vi "UpdateBufferForMultiListBoxIfNecessary.vi"(7 "control refs":T2, 8 "error in":errorcluster, 9 "Buffer Configuration":T3, 10 "TDMS File Viewer Configuration":T3, 11 "TDMS descriptor array":T1(array[cluster])) -> (0 "error out":errorcluster, 1 "BufferConfig out":T3, 3 "TDMS descriptor array out":T1(array[cluster]))   [LabVIEW 2015]
uses:
  <vilib>/Utility/tdmsutil.llb/fileViewerConfigData.ctl
panel:
  in  "tdms file in":refnum<k34>
  out "tdms file out":refnum<k34>
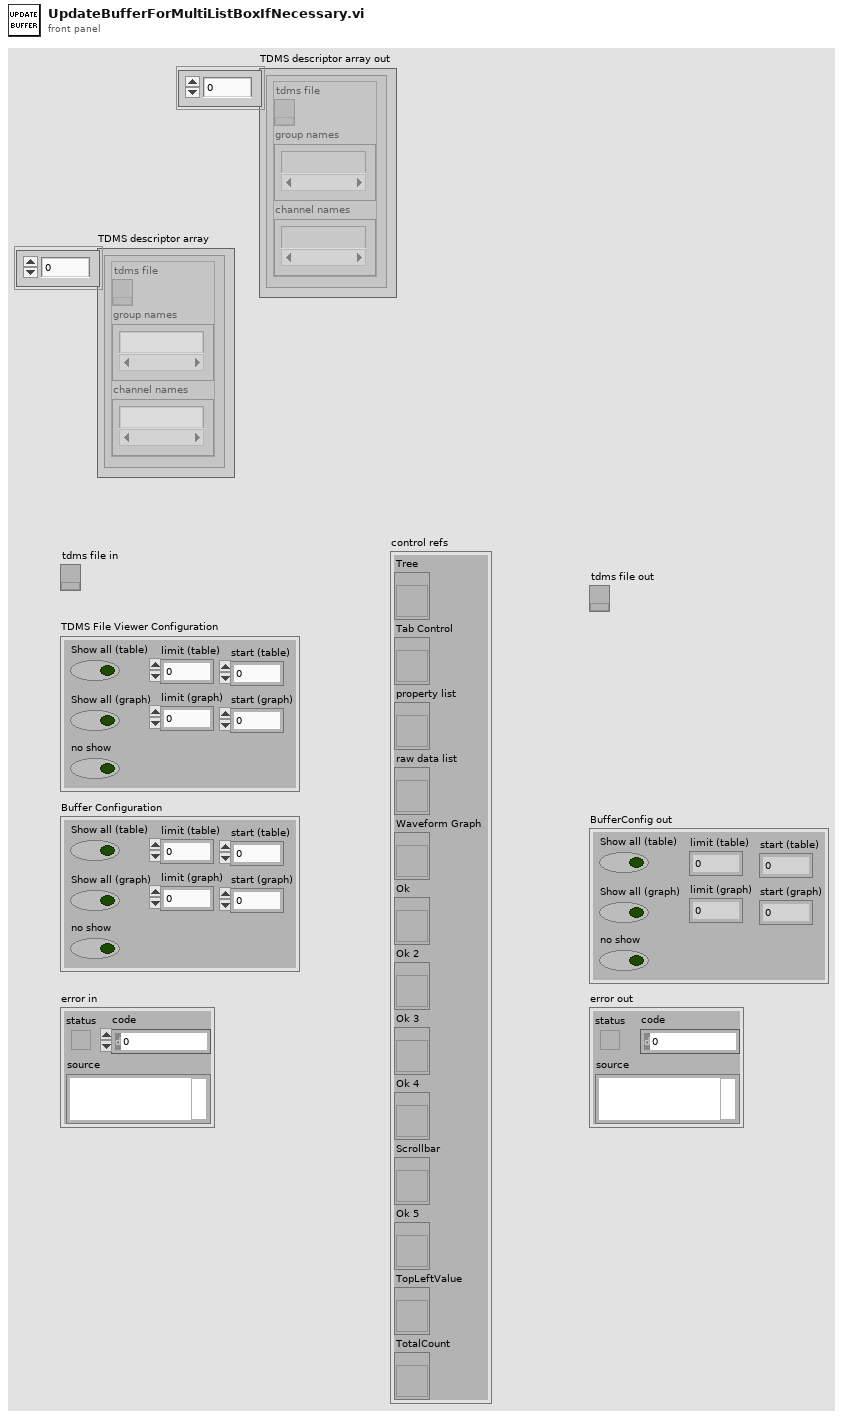
[diagram p1: front panel]
types:
  T1 = cluster{"tdms file ":refnum<k34>, "group names":string[], "channel names":string[]}[]
  T2 = cluster{"Tree":refnum<vi>, "Tab Control":refnum<vi>, "property list":refnum<vi>, "raw data list":refnum<vi>, "Waveform Graph":refnum<vi>, "Ok":refnum<vi>, "Ok 2":refnum<vi>, "Ok 3":refnum<vi>, "Ok 4":refnum<vi>, "Scrollbar":refnum<vi>, "Ok 5":refnum<vi>, "TopLeftValue":refnum<vi>, "TotalCount":refnum<vi>}
  T3 = typedef "fileViewerConfigData.ctl" = cluster{"Show all (table)":bool, "Show all (graph)":bool, "limit (table)":u64, "limit (graph)":u64, "no show":bool, "start (table)":u64, "start (graph)":u64}
  T4 = typedef "LVRowAndColumnUnsignedTypeDef.ctl" = cluster{"Row":u32, "Column":u32}
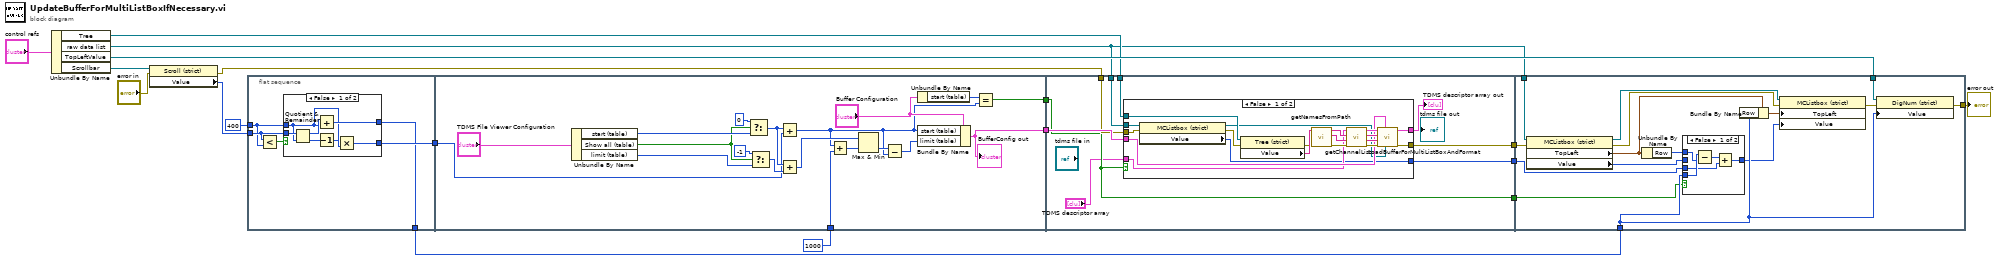
[diagram p0: block diagram]
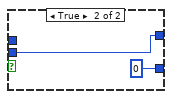
[diagram p2: hidden frame]
diagram:
  n1 = Unbundle By Name("control refs") -> ("Tree"=w8:refnum<vi>, "raw data list"=w7:refnum<vi>, "TopLeftValue"=w16:refnum<vi>, "Scrollbar"=w18:refnum<vi>)
  n2 = property on="Property Node" class="Scroll (strict)"(reference=w18, error in="error in") -> (error out=w9:errorcluster, "Value"=w14:u64)  [unwired: 1 out]
  n3 = flat-sequence {
    tunnel: [w22] -> w15
    tunnel: w14 -> [w21]
    tunnel: [w20] -> w13
    tunnel: u64 400 ("y") -> [w19]
    tunnel: w15 -> [w37]
    tunnel: [w36] -> w12
    tunnel: [w35] -> w11
    tunnel: u64 1000 ("y") -> [w33]
    tunnel: w12 -> [w55]
    tunnel: w11 -> [w60]
    tunnel: [w59] -> w10
    tunnel: w9 -> [w58]
    tunnel: w8 -> [w57]
    tunnel: w7 -> [w56]
    tunnel: [w55] -> w3
    tunnel: [w54] -> w2
    tunnel: w7 -> [w92]
    tunnel: w13 -> [w88]
    tunnel: w16 -> [w91]
    tunnel: w10 -> [w90]
    tunnel: [w89] -> w6
    tunnel: w3 -> [w87]
    tunnel: w2 -> [w86]
    frame #0 {
      n4 = Less?(x=w21, y=w19) -> (x < y?=w23:bool)
      n5 = case shown="False" w23 {
        tunnel: w21 -> [w30 w32]
        tunnel: [w28 w32] -> w20
        tunnel: [w27 u64 0] -> w22
        tunnel: w19 -> [w26 _]
        frame False {
          n6 = Quotient & Remainder(x=w30, y=w26) -> (x-y*floor(x/y)=w29:u64, floor(x/y)=w25:u64)
          n7 = Add(x=w29, y=w26) -> (x+y=w28:u64)
          n8 = Decrement(x=w25) -> (x-1=w24:u64)
          n9 = Multiply(x=w24, y=w26) -> (x*y=w27:u64)
        }
        frame True {
        }
      }
    }
    frame #1 {
      n10 = Unbundle By Name("TDMS File Viewer Configuration") -> ("start (table)"=w45:u64, "Show all (table)"=w38:bool, "limit (table)"=w44:u64)
      n11 = Select(t=u64 0, s=w38, f=w45) -> (s? t:f=w43:u64)
      n12 = Select(t=i64 -1, s=w38, f=w44) -> (s? t:f=w42:u64)
      n13 = Add(x=w43, y=w37) -> (x+y=w34:u64)
      n14 = Add(x=w43, y=w42) -> (x+y=w41:u64)
      n15 = Add(x=w34, y=w33) -> (x+y=w50:u64)
      n16 = Max & Min(x=w41, y=w50) -> (min(x,y)=w49:u64)  [unwired: 1 out]
      n17 = Subtract(x=w49, y=w34) -> (x-y=w48:u64)
      n18 = Unbundle By Name("Buffer Configuration") -> ("start (table)"=w46:u64)
      n19 = Bundle By Name(cluster="Buffer Configuration", "start (table)"=w34, "limit (table)"=w48) -> (w35:T3)
      "BufferConfig out" <- w35
      n20 = Equal?(x=w46, y=w34) -> (x = y?=w36:bool)
    }
    frame #2 {
      n21 = case shown="False" w55 {
        tunnel: [w75 w81] -> w59
        tunnel: [w70 w80] -> w52
        tunnel: w60 -> [w69 _]
        tunnel: w57 -> [w68 _]
        tunnel: w58 -> [w64 w81]
        tunnel: w56 -> [w65 _]
        tunnel: "TDMS descriptor array" -> [w66 w80]
        tunnel: [w61 _] -> w54
        frame False {
          n22 = property on="Property Node" class="MCListbox (strict)"(reference=w65, error in=w64) -> (reference out=w63:refnum<vi>, error out=w62:errorcluster, "Value"=w61:i32)
          n23 = property class="Tree (strict)"(reference=w68, error in=w62) -> (error out=w67:errorcluster, "Value"=w79:string)  [unwired: 1 out]
          n24 = call "getNamesFromPath.vi"("error in (no error)"=w67, "tree path"=w79) -> ("error out"=w78:errorcluster, "channel"=w76:string, "group"=w77:string)  [unwired: 1 in, 2 out]
          n25 = call "getChannelList.vi"("error in (no error)"=w78, "channel names"=w76, "group name"=w77, "TDMS descriptor array"=w66) -> ("error out"=w74:errorcluster, "channel names out"=w73:string[], "group names out"=w72:string[], "TDMS descriptor array out"=w71:T1)
          n26 = call "LoadBufferForMultiListBoxAndFormat.vi"("MCListbox Refnum"=w63, "configuration in"=w69, "error in (no error)"=w74, "channel names in"=w73, "group names in"=w72, "TDMS descriptor array"=w71) -> ("error out"=w75:errorcluster, "TDMS descriptor array out"=w70:T1)  [unwired: 4 in]
        }
        frame True {
        }
      }
      "TDMS descriptor array out" <- w52
    }
    frame #3 {
      n27 = property on="Property Node" class="MCListbox (strict)"(reference=w92, error in=w90) -> (reference out=w93:refnum<vi>, error out=w95:errorcluster, "TopLeft"=w84:T4, "Value"=w85:i32)
      n28 = Unbundle By Name(w84) -> ("Row"=w83:u32)
      n29 = case shown="False" w87 {
        tunnel: [w101 w102] -> w82
        tunnel: w88 -> [w100 _]
        tunnel: w86 -> [w97 _]
        tunnel: w85 -> [_ w102]
        tunnel: w83 -> [w99 _]
        frame False {
          n30 = Subtract(x=w100, y=w99) -> (x-y=w98:u64)
          n31 = Add(x=w98, y=w97) -> (x+y=w101:u64)
        }
        frame True {
        }
      }
      n32 = Bundle By Name(cluster=w84, "Row"=w88) -> (w94:T4)
      n33 = property on="Property Node" class="MCListbox (strict)"(reference=w93, error in=w95, "TopLeft"=w94, "Value"=w82) -> (error out=w96:errorcluster)  [unwired: 1 out]
      n34 = property on="Property Node" class="DigNum (strict)"(reference=w91, error in=w96, "Value"=w88) -> (error out=w89:errorcluster)  [unwired: 1 out]
    }
  }
  "error out" <- w6
